vi "Empty Port.vi"(8 "entrée d'erreur (pas d'erreur)":errorcluster, 11 "Send_Frame en entrée":refnum<class "Nodon_Send_Command_UART.lvclass">) -> (0 "sortie d'erreur":errorcluster, 3 "Send_Frame en sortie":refnum<class "Nodon_Send_Command_UART.lvclass">)   [LabVIEW 2020, in "Library Test.lvlib" / "Nodon_Send_Command_UART.lvclass"]
uses:
  Nodon_Send_Command_UART.lvclass
  C:/Users/ngarcin/OneDrive - Altyor/Standard TB/Class/Test/Test (Default)/Test (Default).lvclass
  Commun VI/TypeDef/Commande UART/Parametre UART.ctl
  UART/UART (Default)/Class UART (Default).lvclass
  JSON API/JSON Value/Set from JSON string.vi
  Instrument/Instrument (Default)/Class Instrument (Default).lvclass
  JSON API/JSON Value/JSON Value.lvclass
  Nodon_Send_Command_UART.lvclass/Nodon_Send_Command_UART.ctl
  JSON API/Variant JSON/Variant JSON.lvlib
  JSON API/Get Polymorphic/JSON GetSet.lvlib
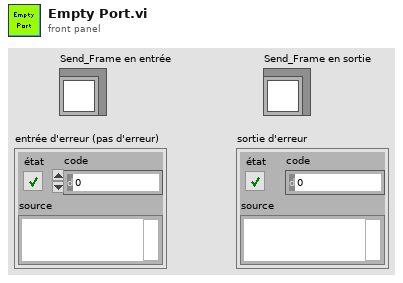
[diagram p1: front panel]
types:
  T1 = typedef "Parametre UART.ctl" = cluster{"Address Device":refnum<visa-resource-name>, "Baud Rate":u32, "Data Bit":u16, "stop bits (10: 1 bit)":u16, "parity (0:none)":enum16{"None", "Odd", "Even", "Mark", "Space"}, "flow control (0:none)":u16, "termination char ":u8, "Enable Termination":bool, "Nb Octet to Read":u16, "Class UART":refnum<class "Class UART (Default).lvclass">}
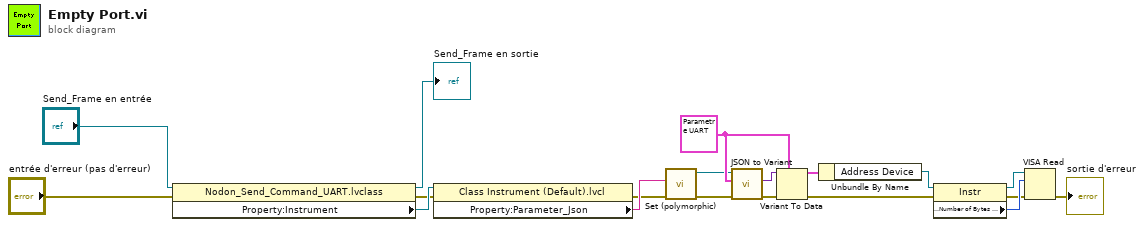
[diagram p0: block diagram]
diagram:
  w17 = T1 {"Address Device"="", "Baud Rate"=0, "Data Bit"=0, "stop bits (10: 1 bit)"=0, "parity (0:none)"=enum."None", "flow control (0:none)"=0, "termination char "=0, "Enable Termination"=FALSE, "Nb Octet to Read"=0, "Class UART"=refnum} ("Parameter")
  n1 = property class="Nodon_Send_Command_UART.lvclass"(reference="Send_Frame en entrée", error in="entrée d'erreur (pas d'erreur)") -> (reference out=→"Send_Frame en sortie":refnum<class "Nodon_Send_Command_UART.lvclass">, error out=w2:errorcluster, "Property:Instrument"=w4:refnum<class "Class Instrument (Default).lvclass">)
  n2 = property class="Class Instrument (Default).lvcl"(reference=w4, error in=w2) -> (error out=w12:errorcluster, "Property:Parameter_Json"=w18:string)  [unwired: 1 out]
  n3 = call-poly "Set (polymorphic).vi"("error in (no error)"=w12, "JSON stream"=w18) -> ("error out"=w15:errorcluster, "JSON Value out"=w13:refnum<class "JSON Value.lvclass">)  [unwired: 7 in, 1 out]
  n4 = call "JSON to Variant.vi"("error in (no error)"=w15, "Variant (Data Type)"=w17, "JSON Value"=w13) -> ("error out"=w14:errorcluster, "Variant out"=w16:variant)  [unwired: 7 in]
  n5 = Variant To Data(error in=w14, type=w17, Variant=w16) -> (data=w19:T1, error out=w7:errorcluster)
  n6 = Unbundle By Name(w19) -> ("Address Device"=w11:refnum<visa-resource-name>)
  n7 = property class="Instr"(reference=w11, error in=w7) -> (reference out=w9:refnum<visa-resource-name>, error out=w8:errorcluster, "Serial Settings:Number of Bytes at Serial Port"=w10:u32)
  n8 = VISA Read(VISA resource name=w9, byte count=w10, error in (no error)=w8) -> (error out=→"sortie d'erreur":errorcluster)  [unwired: 3 out]
